vi "save_ctab.vi"(5 "Array":cluster{"Uin":dbl[], "ADCode":dbl[]}[](array[cluster]), 7 "path":path) -> ()   [LabVIEW 2010]
uses:
  <vilib>/Utility/xml.llb/Write to XML File(string).vi
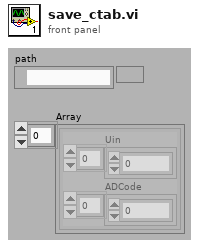
[diagram p1: front panel]
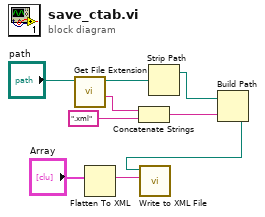
[diagram p0: block diagram]
diagram:
  n1 = call <vilib>:"Get File Extension.vi"("file"="path") -> ("filename without extension"=w6:string, "dup file"=w4:path)  [unwired: 7 in, 2 out]
  n2 = Flatten To XML(anything="Array") -> (xml string=w1:string)
  n3 = Concatenate Strings(w6, ".xml" ("string")) -> (w8:string)
  n4 = Strip Path(path=w4) -> (stripped path=w5:path)  [unwired: 1 out]
  n5 = Build Path(base path=w5, name or relative path=w8) -> (appended path=w9:path)
  n6 = call-poly <vilib>:"Write to XML File.vi"("XML Input"=w1, "XML File Path"=w9) -> ()  [unwired: 7 in, 3 out]
